vi "TpUSBEventLevel1.vi"() -> (1 "TracepointName":string)   [LabVIEW 2017, in "USBDrive.lvlib"]
uses:
  <vilib>/addons/InsightCM/Devices/Shared/Common/USBDrive/USBDrive.lvlib
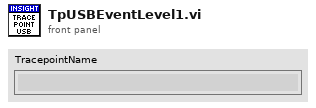
[diagram p1: front panel]
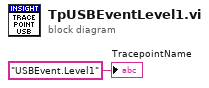
[diagram p0: block diagram]
diagram:
  "TracepointName" <- "USBEvent.Level1" ("ProcessName")
